vi "Dispose.vi"(8 "error in (no error)":errorcluster, 11 "Data Value Reference in":refnum<data-value>) -> (0 "error out":errorcluster)   [LabVIEW 2020, in "Progress Bar.lvclass"]
doc: "Deletes the reference\n\nCopyright: MGI\nAuthored by: Derek Trepanier"
uses:
  <userlib>/_MGI/User Interface/Progress Bar/Progress Bar.lvclass
  <userlib>/_MGI/User Interface/Progress Bar/Progress Bar.lvclass/Progress Bar.ctl
  <userlib>/_MGI/User Interface/Progress Bar/Progress Bar Settings/Progress Bar Settings.lvclass
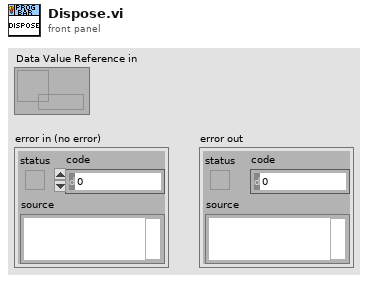
[diagram p1: front panel]
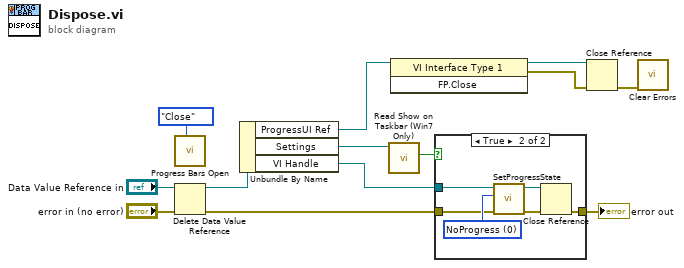
[diagram p0: block diagram]
diagram:
  n1 = call <userlib>:"Progress Bars Open.vi"("Method"=enum16{"Open New", "Close", "Get"}."Close") -> ()  [unwired: 10 in, 1 out]
  n2 = Delete Data Value Reference(data value reference="Data Value Reference in", error in="error in (no error)") -> (data value=w10:refnum<class "Progress Bar.lvclass">, error out=w3:errorcluster)
  n3 = Unbundle By Name(w10) -> ("ProgressUI Ref"=w13:refnum<vi>, "Settings"=w8:refnum<class "Progress Bar Settings.lvclass">, "VI Handle"=w2:refnum<k24>)
  n4 = call-dynamic "Read Show on Taskbar (Win7 Only).vi"("MGI_Progress Bar Options in"=w8) -> ("Show on Taskbar (Win7 Only)"=w7:bool)  [unwired: 8 in, 2 out]
  n5 = invoke class="VI Interface Type 1" method="FP.Close"(reference=w13) -> (reference out=w9:refnum<vi>, error out=w5:errorcluster)  [unwired: 2 in, 1 out]
  n6 = case shown="True" w7 {
    tunnel: w2 -> [_ w18]
    tunnel: w3 -> [w14 w17]
    tunnel: [w14 w20] -> w1
    frame False {
    }
    frame True {
      w19 = 0 items=["NoProgress"=0, "Indeterminate"=1, "Normal"=2, "Error"=4, "Paused"=8] ("State (No Progress)")
      n7 = call <userlib>:"SetProgressState.vi"("error in (no error)"=w17, "State (No Progress)"=w19, "Window Handle"=w18) -> ("error out"=w15:errorcluster, "dup Window Handle"=w16:refnum<k24>)  [unwired: 7 in]
      n8 = Close Reference(reference=w16, error in (no error)=w15) -> (error out=w20:errorcluster)
    }
  }
  "error out" <- w1
  n9 = Close Reference(reference=w9, error in (no error)=w5) -> (error out=w6:errorcluster)
  n10 = call <vilib>:"Clear Errors.vi"("error in (no error)"=w6) -> ()  [unwired: 5 in, 2 out]
